vi "TCP Server.vi"() -> ()   [LabVIEW 2020]
panel:
  in  "Remote Server name":string
  in  "remote port or service name":u16
  in  "error in (no error)":errorcluster
  out "bytes written":i32
  in  "abort (F)":bool
  in  "string 2":string
  in  "string":string
  out "error out":errorcluster
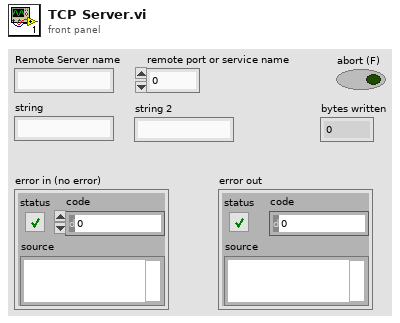
[diagram p1: front panel]
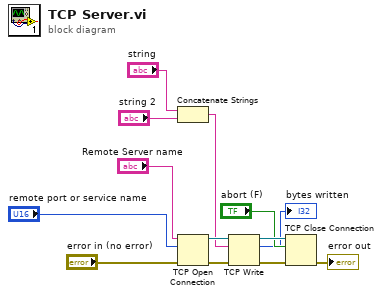
[diagram p0: block diagram]
diagram:
  n1 = Concatenate Strings("string", "string 2") -> (w8:string)
  n2 = TCP Open Connection(address="Remote Server name", remote port or service name="remote port or service name", error in (no error)="error in (no error)") -> (connection ID=w9:refnum<k5>, error out=w13:errorcluster)  [unwired: 2 in]
  n3 = TCP Write(connection ID=w9, data in=w8, error in (no error)=w13) -> (connection ID out=w10:refnum<k5>, bytes written=→"bytes written":i32, error out=w12:errorcluster)  [unwired: 1 in]
  n4 = TCP Close Connection(connection ID=w10, abort (F)="abort (F)", error in (no error)=w12) -> (error out=→"error out":errorcluster)  [unwired: 1 out]
